vi "FlatToRichni_bus_monitor_api_InitializeSettingsReply.vi"(5 "OutputClusterType":T1, 11 "InputCluster":T4) -> (3 "OutputCluster":T1)   [LabVIEW 2025, in "bus_monitor_client.lvlib"]
uses:
  bus_monitor_client.lvlib
  ni_bus_monitor_api_InitializeSettingsReply_Flat.ctl
  ni_bus_monitor_api_Session_Flat.ctl
  ni_bus_monitor_api_ErrorInfo_Flat.ctl
  ni_bus_monitor_api_InitializeSettingsReply.ctl
  ni_bus_monitor_api_Session.ctl
  ni_bus_monitor_api_ErrorInfo.ctl
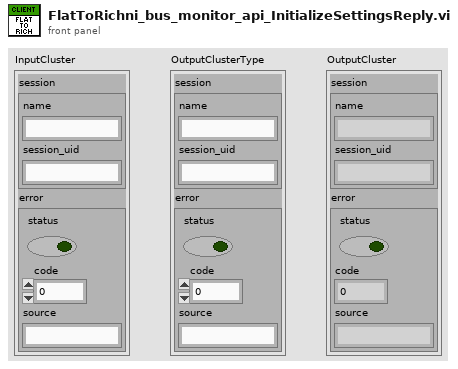
[diagram p1: front panel]
types:
  T1 = typedef "bus_monitor_client.lvlib/ni_bus_monitor_api_InitializeSettingsReply.ctl" = cluster{"session":T2, "error":T3}
  T2 = typedef "bus_monitor_client.lvlib/ni_bus_monitor_api_Session.ctl" = cluster{"name":string, "session_uid":string}
  T3 = typedef "bus_monitor_client.lvlib/ni_bus_monitor_api_ErrorInfo.ctl" = errorcluster
  T4 = typedef "bus_monitor_client.lvlib/ni_bus_monitor_api_InitializeSettingsReply_Flat.ctl" = cluster{"session":T5, "error":T6}
  T5 = typedef "bus_monitor_client.lvlib/ni_bus_monitor_api_Session_Flat.ctl" = cluster{"name":string, "session_uid":string}
  T6 = typedef "bus_monitor_client.lvlib/ni_bus_monitor_api_ErrorInfo_Flat.ctl" = errorcluster
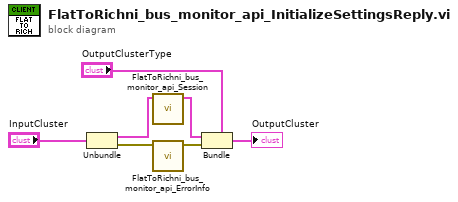
[diagram p0: block diagram]
diagram:
  n1 = Unbundle "Unbundle"("InputCluster") -> ("session"=w4:T5, "error"=w2:T6)
  n2 = call "FlatToRichni_bus_monitor_api_Session.vi"("InputCluster"=w4) -> ("OutputCluster"=w3:T2)  [unwired: 10 in]
  n3 = call "FlatToRichni_bus_monitor_api_ErrorInfo.vi"("InputCluster"=w2) -> ("OutputCluster"=w1:T3)  [unwired: 10 in]
  n4 = Bundle "Bundle"(cluster="OutputClusterType", "session"=w3, "error"=w1) -> (→"OutputCluster":T1)
